vi "test_SessionsRegistered_ReserveRegisteredSessions_ReservesAllSessions.vi"(8 "error in":errorcluster) -> (0 "error out":errorcluster, 2 "result":string, 3 "pass":bool)   [LabVIEW 2020, in "MeasurementServerTests.lvlib" / "Session Reservation Tests.lvlib"]
uses:
  Session Reservation Tests.lvlib
  MeasurementServerTests.lvlib
  Runtime/APIs/Session Management V1/Session Reservation/Session Reservation.lvclass
  TestUtilities/TestUtilities.Runtime/Session Reservation Test Utilities/Session Reservation Test Utilities.lvlib
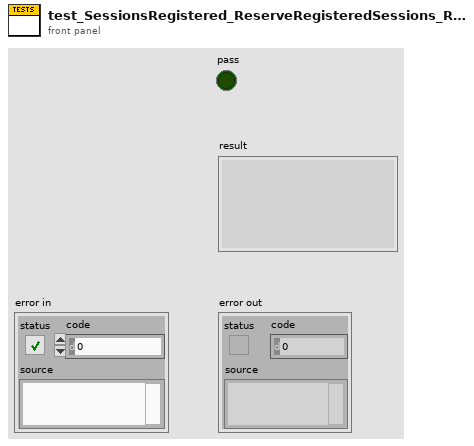
[diagram p1: front panel]
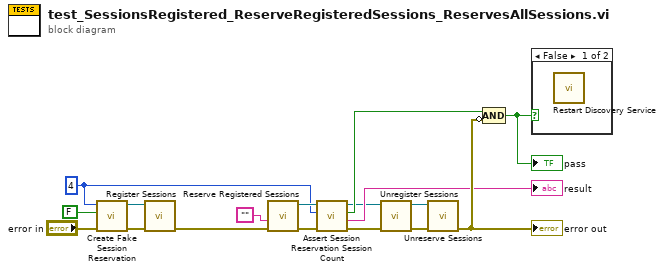
[diagram p0: block diagram]
diagram:
  w6 = 4 ("number of sessions")
  n1 = call "Create Fake Session Reservation.vi"("error in"="error in", "session exists"=FALSE, "number of sessions"=w6) -> ("error out"=w12:errorcluster, "session reservation out"=w11:refnum<class "Session Reservation.lvclass">)  [unwired: 7 in]
  n2 = call "Register Sessions.vi"("error in"=w12, "session reservation in"=w11) -> ("error out"=w9:errorcluster)  [unwired: 8 in, 1 out]
  n3 = call "Reserve Registered Sessions.vi"("error in"=w9, "instrument type id"="") -> ("error out"=w5:errorcluster, "session reservation out"=w7:refnum<class "Session Reservation.lvclass">)  [unwired: 8 in]
  n4 = call "Assert Session Reservation Session Count.vi"("error in"=w5, "expected value"=w6, "session reservation in"=w7) -> ("error out"=w4:errorcluster, "result"=→"result":string, "pass"=w3:bool, "session reservation out"=w1:refnum<class "Session Reservation.lvclass">)  [unwired: 5 in]
  n5 = call "Unregister Sessions.vi"("error in"=w4, "session reservation in"=w1) -> ("error out"=w15:errorcluster, "session reservation out"=w14:refnum<class "Session Reservation.lvclass">)  [unwired: 8 in]
  n6 = call "Unreserve Sessions.vi"("error in"=w15, "session reservation in"=w14) -> ("error out"=w17:errorcluster)  [unwired: 9 in]
  "error out" <- w17
  n7 = Compound Arithmetic op=AND(w3, invert w17) -> (w16:bool)
  "pass" <- w16
  n8 = case shown="False" w16 {
    frame False {
      n9 = call "Restart Discovery Service.vi"() -> ()  [unwired: 11 in, 1 out]
    }
    frame True {
    }
  }
